vi "G#Object_Open.vi"(0 "reference in":refnum<class "G#Interface.lvclass">, 5 "error in (no error)":errorcluster) -> (14 "reference out":refnum<class "G#Interface.lvclass">, 19 "error out":errorcluster)   [LabVIEW 2017, in "G#Interface.lvclass"]
doc: "Dummy VI to define the interface of the G#Object_Open method. This method could be executed by the External Create Process (if running)."
uses:
  <vilib>/addons/_AddQ/G#Interface/G#Interface.lvclass
  <vilib>/addons/_AddQ/G#Interface/G#Interface.lvclass/G#Interface.ctl
  <vilib>/addons/_AddQ/G#Object/G#Object.lvclass
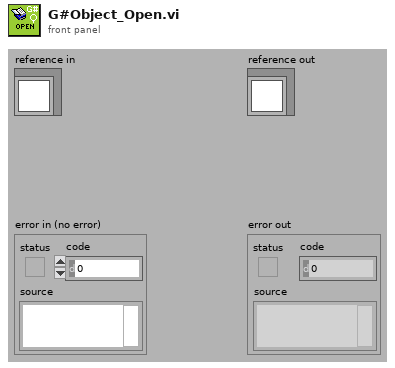
[diagram p1: front panel]
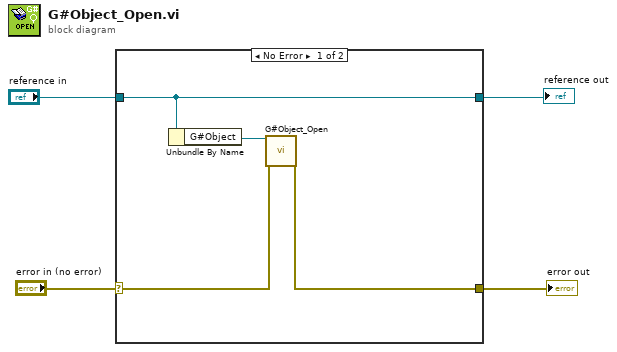
[diagram p0: block diagram]
diagram:
  n1 = case shown="No Error" "error in (no error)" {
    selector: "error in (no error)" -> [w6 w9]
    tunnel: "reference in" -> [w5 w10]
    tunnel: [w7 w9] -> w3
    tunnel: [w5 w10] -> w1
    frame No Error {
      n2 = Unbundle By Name(w5) -> ("G#Object"=w8:refnum<class "G#Object.lvclass">)
      n3 = call-dynamic "G#Object_Open.vi"("reference in"=w8, "error in (no error)"=w6) -> ("error out"=w7:errorcluster)  [unwired: 16 in, 1 out]
    }
    frame Error {
    }
  }
  "error out" <- w3
  "reference out" <- w1
